vi "Tek.vi"() -> ()   [LabVIEW 2016]
panel:
  out "错误输出":errorcluster caption="连接状态"
  in  "查询":bool
  in  "写入":bool
  in  "历史记录":string
  in  "命令":string
  in  "VISA资源名称":refnum<visa-resource-name>
  in  "连接":bool
  out "外循环":i32
  out "内循环":i32
  in  "停止":bool
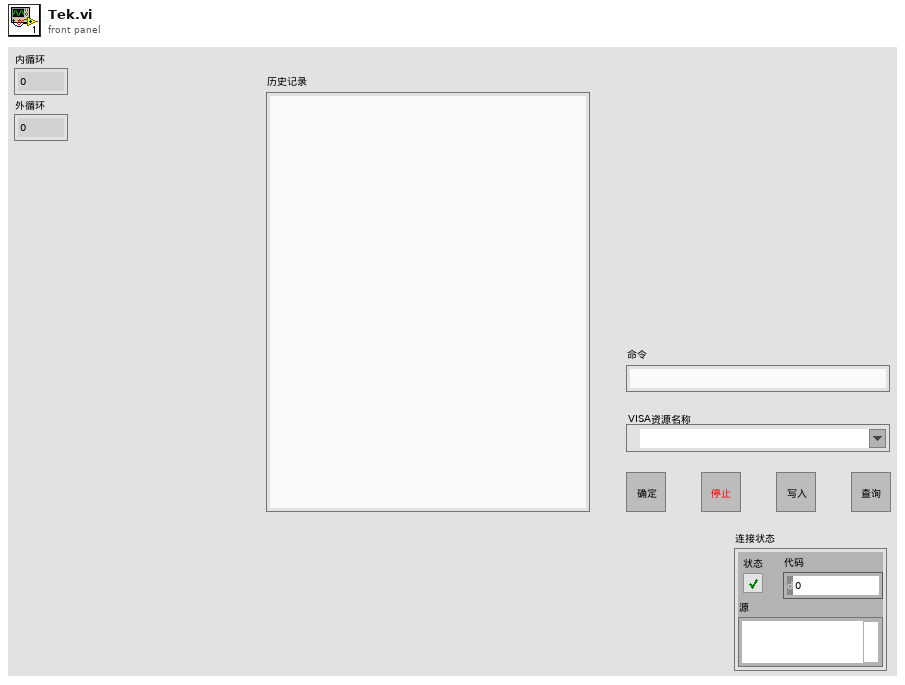
[diagram p1: front panel]
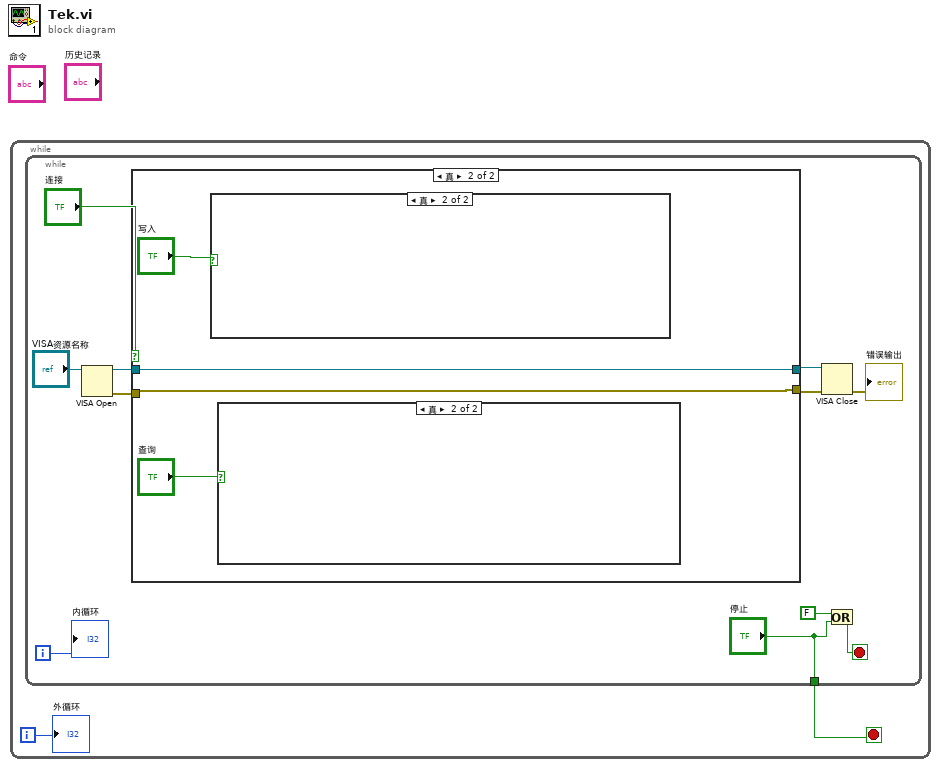
[diagram p0: block diagram]
diagram:
  n1 = while {
    i -> [w1]
    stop <- w2 stop-if-true
    n2 = while {
      tunnel: ["停止"] -> w2
      i -> [w13]
      stop <- w5 stop-if-true
      n3 = VISA Open(VISA resource name="VISA资源名称") -> (VISA resource name=w8:refnum<visa-resource-name>, error out=w7:errorcluster)  [unwired: 4 in]
      n4 = case shown="真" "连接" {
        tunnel: [w15 w17] -> w9
        tunnel: w8 -> [w15 w17]
        tunnel: [w14 w16] -> w6
        tunnel: w7 -> [w14 w16]
        frame False {
        }
        frame True {
          n5 = case shown="真" "写入" {
            frame False {
            }
            frame True {
            }
          }
          n6 = case shown="真" "查询" {
            frame False {
            }
            frame True {
            }
          }
        }
      }
      n7 = VISA Close(VISA resource name=w9, error in (no error)=w6) -> (error out=→"错误输出":errorcluster)
      n8 = Or(x=FALSE, y="停止") -> (x .or. y?=w5:bool)
      "内循环" <- w13
    }
    "外循环" <- w1
  }
